vi "Wait for DRDY.vi"(8 "error in (no error)":errorcluster, 10 "Timeout (1000ms)":u32=1000, 11 "LINX-ADS1256 in":refnum<class "LINX-ADS1256.lvclass">) -> (0 "error out":errorcluster, 1 "Wait Time (ms)":u32, 2 "DRDY":bool, 3 "LINX-ADS1256 out":refnum<class "LINX-ADS1256.lvclass">)   [LabVIEW 2020, in "LINX-ADS1256.lvclass"]
doc: "Wait for DRDY (data ready) bit from the status register to be low."
uses:
  LINX-ADS1256.lvclass
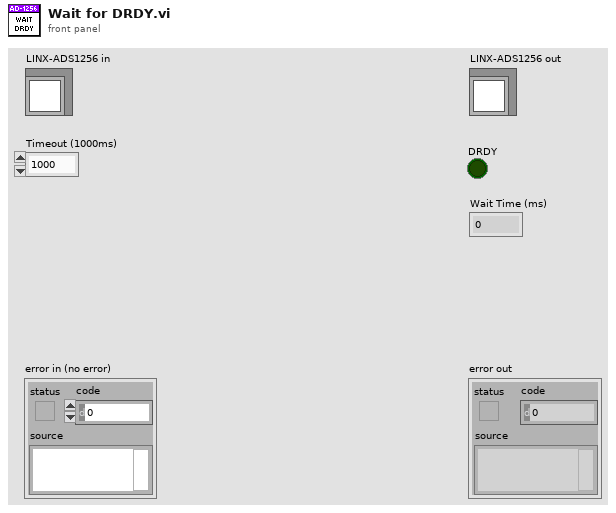
[diagram p1: front panel]
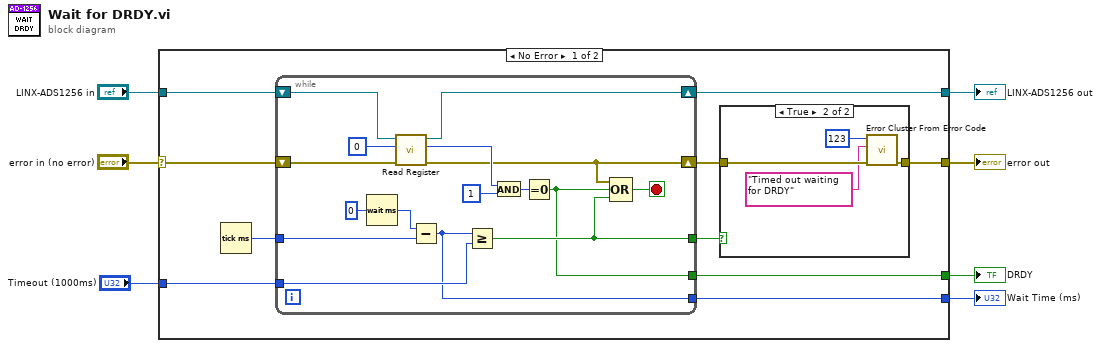
[diagram p0: block diagram]
diagram:
  n1 = case shown="No Error" "error in (no error)" {
    selector: "error in (no error)" -> [w16 w40]
    tunnel: [w12 w40] -> w6
    tunnel: [w15 w39] -> w4
    tunnel: "LINX-ADS1256 in" -> [w17 w39]
    tunnel: "Timeout (1000ms)" -> [w10 _]
    tunnel: [w9 _] -> w2
    tunnel: [w8 _] -> w1
    frame No Error {
      n2 = Tick Count (ms)() -> (millisecond timer value=w14:u32)
      n3 = while {
        shift-right: [w32] -> w15
        shift-left: w17 -> [w38]
        shift-right: [w31] -> w13
        shift-left: w16 -> [w37]
        tunnel: w14 -> [w27]
        tunnel: [w26] -> w11
        tunnel: w10 -> [w25]
        tunnel: [w24] -> w9
        tunnel: [w23] -> w8
        stop <- w30 stop-if-true
        n4 = Wait (ms)(milliseconds to wait=u32 0) -> (millisecond timer value=w28:u32)
        n5 = call "Read Register.vi"("error in (no error)"=w37, "Register Address"=u8 0, "LINX-ADS1256 in"=w38) -> ("error out"=w31:errorcluster, "Read Data"=w35:u8, "LINX-ADS1256 out"=w32:refnum<class "LINX-ADS1256.lvclass">)  [unwired: 6 in]
        n6 = Subtract(x=w28, y=w27) -> (x-y=w24:u32)
        n7 = Greater Or Equal?(x=w24, y=w25) -> (x >= y?=w26:bool)
        n8 = And(x=w35, y=u8 1) -> (x .and. y?=w33:u8)
        n9 = Equal To 0?(x=w33) -> (x = 0?=w23:bool)
        n10 = Compound Arithmetic op=OR(w31, w23, w26) -> (w30:bool)
      }
      n11 = case shown="True" w11 {
        tunnel: w13 -> [w18 w22]
        tunnel: [w18 w21] -> w12
        frame False {
        }
        frame True {
          n12 = call <vilib>:"Error Cluster From Error Code.vi"("error in (no error)"=w22, "error message (\"\")"="Timed out waiting for DRDY", "error code (0)"=123) -> ("error out"=w21:errorcluster)  [unwired: 6 in]
        }
      }
    }
    frame Error {
    }
  }
  "error out" <- w6
  "LINX-ADS1256 out" <- w4
  "Wait Time (ms)" <- w2
  "DRDY" <- w1
